vi "VI Server_TREE_Column_Color_SET.vi"(4 "BG.Color":u32(colorbox), 6 "Active Cell:Active Column Number":i32=3, 7 "Label":string, 8 "error in":errorcluster, 9 "Tree.Ref":refnum<vi>, 11 "VI Server.RefsCluster":T1) -> (0 "error out":errorcluster, 1 "Tree.Ref.DUP":refnum<vi>, 3 "VI Server.RefsCluster.DUP":T1)   [LabVIEW 2020]
uses:
  VI Server_TypeDefs/VI Server_RefsCluster.ctl
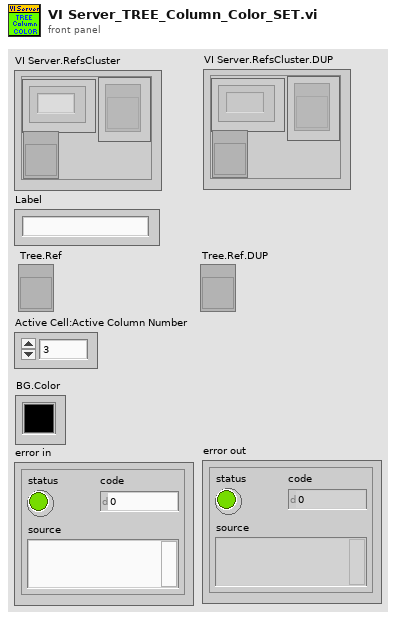
[diagram p1: front panel]
types:
  T1 = typedef "VI Server_RefsCluster.ctl" = cluster{"Labels":string[], "Refs":refnum<vi>[], "VI Ref":refnum<vi>}
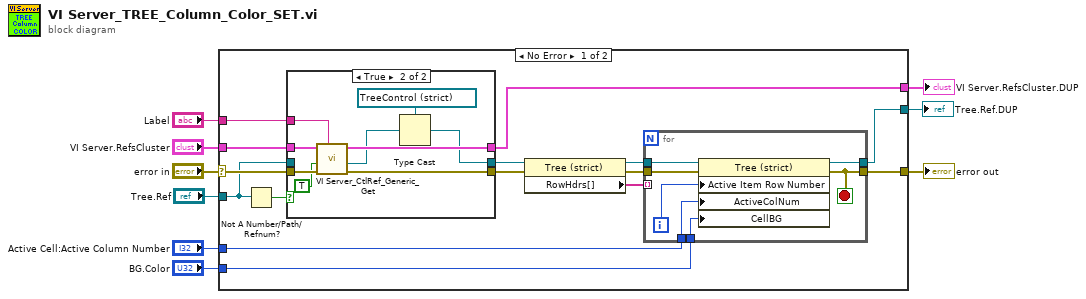
[diagram p0: block diagram]
diagram:
  n1 = case shown="No Error" "error in" {
    selector: "error in" -> [w24 w45]
    tunnel: [w18 w45] -> w8
    tunnel: "VI Server.RefsCluster" -> [w23 w44]
    tunnel: [w22 w44] -> w6
    tunnel: "Label" -> [w21 _]
    tunnel: [w17 _] -> w1
    tunnel: "Tree.Ref" -> [w19 _]
    tunnel: "Active Cell:Active Column Number" -> [w11 _]
    tunnel: "BG.Color" -> [w16 _]
    frame No Error {
      n2 = Not A Number/Path/Refnum?(number/path/refnum=w19) -> (NaN/Path/Refnum?=w20:bool)
      n3 = case shown="True" w20 {
        tunnel: w24 -> [w34 w43]
        tunnel: w23 -> [w32 w42]
        tunnel: [w32 w41] -> w22
        tunnel: w21 -> [_ w40]
        tunnel: [w33 w38] -> w13
        tunnel: [w34 w37] -> w15
        tunnel: w19 -> [w33 _]
        frame False {
        }
        frame True {
          n4 = call "VI Server_CtlRef_Generic_Get.vi"("Control.Label"=w40, "error in"=w43, "SingleInstance"=TRUE, "VI Server.RefsCluster"=w42) -> ("error out"=w37:errorcluster, "Control.Ref.Generic"=w39:refnum<vi>, "VI Server.RefsCluster.DUP"=w41:T1)  [unwired: 5 in]
          n5 = Type Cast(type=refnum<vi> refnum ("Test.Tree"), x=w39) -> (*(type *) &x=w38:refnum<vi>)
        }
      }
      n6 = property on="Property Node" class="Tree (strict)"(reference=w13, error in=w15) -> (reference out=w12:refnum<vi>, error out=w14:errorcluster, "RowHdrs[]"=w10:string[])
      n7 = for {
        tunnel: w16 -> [w30]
        tunnel: w11 -> [w27]
        tunnel: w14 -> [w29]
        tunnel: [w26] -> w18
        tunnel: w12 -> [w28]
        tunnel: [w31] -> w17
        tunnel: w10 -> [_] mode=indexing
        i -> [w25]
        stop <- w26 stop-if-true
        n8 = property on="Property Node" class="Tree (strict)"(reference=w28, error in=w29, "Active Item Row Number"=w25, "ActiveColNum"=w27, "CellBG"=w30) -> (reference out=w31:refnum<vi>, error out=w26:errorcluster)
      }
    }
    frame Error {
    }
  }
  "VI Server.RefsCluster.DUP" <- w6
  "error out" <- w8
  "Tree.Ref.DUP" <- w1
